vi "ROI Stand Alone Compatability check.vi"(8 "error in (no error)":errorcluster, 11 "Old ROI file path":path) -> (0 "error out":errorcluster, 1 "Proceed":bool, 3 "ROI file path (dup)":path, 5 "ROI fit info cluster":T1 {"ROI fit info"."Frame size"."Old" items=["100X100"=100, "128X128"=128, "200X200"=200, "256X256"=256, "512X512"=512, "1024x1024"=1024, "2048x2048"=2048]; "ROI fit info"."Frame size"."New" items=["100X100"=100, "128X128"=128, "200X200"=200, "256X256"=256, "512X512"=512, "1024x1024"=1024, "2048x2048"=2048]})   [LabVIEW 2017]
uses:
  Typedefs/ROI fitting info cluster.ctl
  Typedefs/Frame Size.ctl
  Typedefs/ROI ID Enum.ctl
  Typedefs/ROI management FG states.ctl
  <userlib>/My Palettes.lib/Files & paths/Spreadsheet/Read From Spreadsheet File (DBL)-Mod.vi
  Globals/gl_ROI Entry UI globals.vi
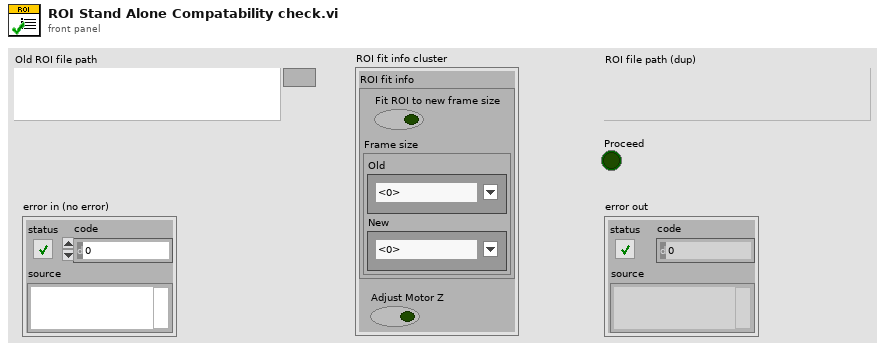
[diagram p1: front panel]
types:
  T1 = typedef "ROI fitting info cluster.ctl" = cluster{"ROI fit info":cluster{"Fit ROI to new frame size":bool, "Frame size":cluster{"Old":T2, "New":T2}}, "Adjust Motor Z":bool}
  T2 = typedef "Frame Size.ctl" = u16
  T3 = typedef "Fixed strings.ctl" = cluster{"ROI file name":string, "Normalised ROI file name":string, "Zplane Pockels values file name":string, "Functional data folder name":string, "Experiment Header file name":string, "Z-stack images folder name":string, "Groups setup rel. path":string, "Groups text file rel. path":string, "TDMS files folder name (F.img)":string, "TDMS files folder name (V.acq)":string, "TDMS files folder name (Pl.acq)":string, "Cycle rel times sequence file":string, "Dynamically called VIs folder name":string, "Time Series folder base name":string}
  T4 = typedef "ROI ID Enum.ctl" = enum16{"Point", "MiniScan", "Comp. MiniScan", "Rectangle", "Comp. volume", "Arb. plane point", "None"}
  T5 = typedef "ROI management FG states.ctl" = enum16{"Read", "Write", "Write-from dataset", "Clear Last", "Clear All", "Update ROIs time", "Reload last ROI set", "Offset all ROI", "Offset visible ROI"}
  T6 = enum8{"Enabled", "Disabled", "Disabled and Grayed Out"}
  T7 = typedef "ROI parameters data type.ctl" = cluster{"ROI index":dbl, "ROI ID":dbl, "ROI Time (ns)":dbl, "Pixels in ROI":dbl, "X start":dbl, "Y start":dbl, "Z start":dbl, "X stop":dbl, "Y stop":dbl, "Z stop":dbl, "Angle (deg)":dbl, "Composite ID":dbl, "Number of lines":dbl, "Frame Size":dbl, "Zoom":dbl, "Laser Power (%)":dbl, "ROI group ID":dbl, "Z Plane Idx":i32[], "Z Plane codes":i32[]}
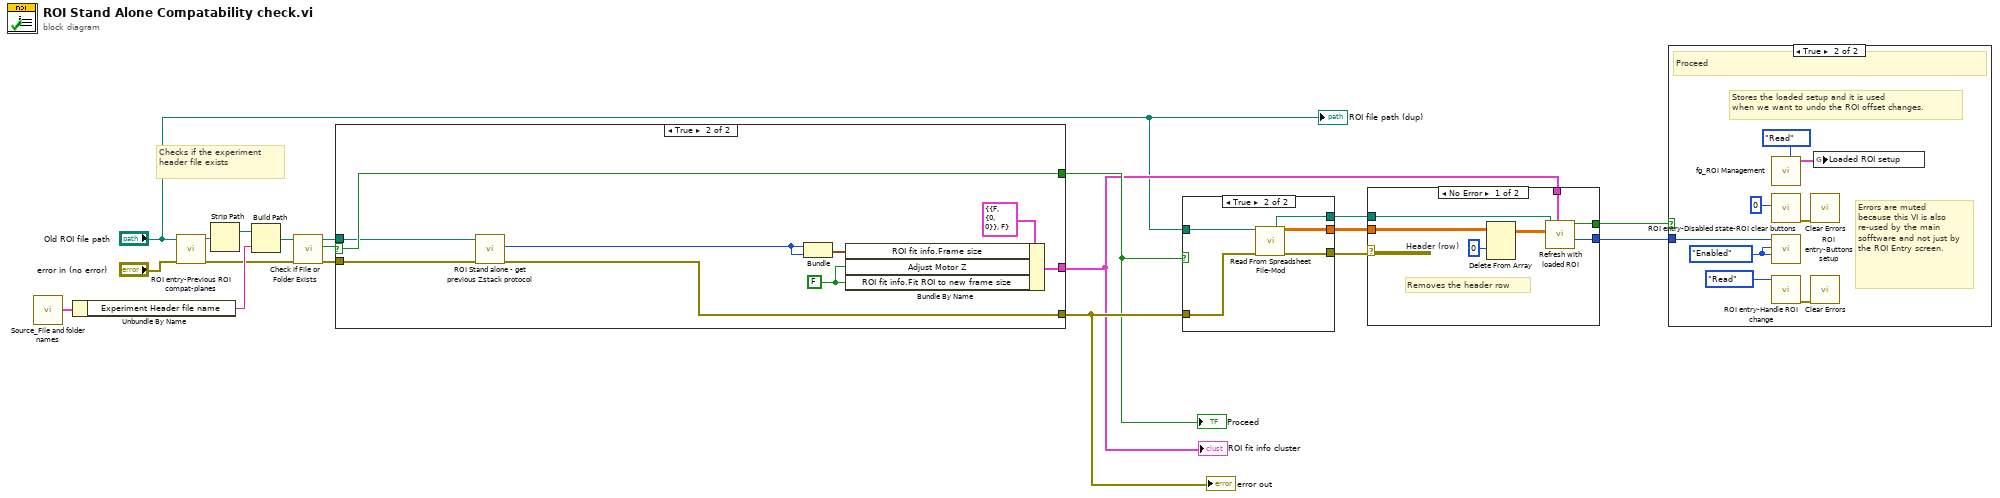
[diagram p0: block diagram]
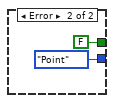
[diagram p3: hidden frame]
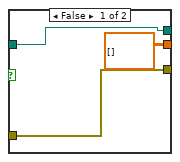
[diagram p4: hidden frame]
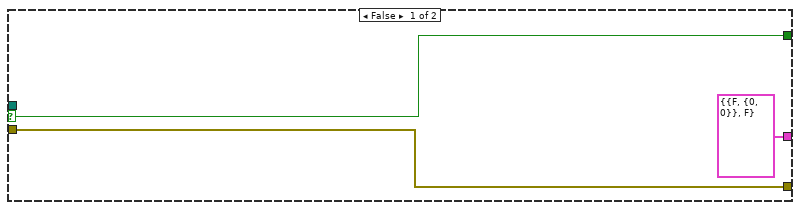
[diagram p5: hidden frame]
diagram:
  # "Checks if the experiment header file exists"
  n1 = call "Source_File and folder names.vi"() -> ("Fixed strings"=w17:T3)  [unwired: 1 in]
  n2 = Unbundle By Name(w17) -> ("Experiment Header file name"=w15:string)
  n3 = call "ROI entry-Previous ROI compat-planes.vi"("error in (no error)"="error in (no error)", "Old ROI file path"="Old ROI file path") -> ("error out"=w14:errorcluster, "Old ROI file path (dup)"=w13:path)  [unwired: 7 in, 1 out]
  n4 = Strip Path(path=w13) -> (stripped path=w16:path)  [unwired: 1 out]
  n5 = Build Path(base path=w16, name or relative path=w15) -> (appended path=w18:path)
  n6 = call <vilib>:"Check if File or Folder Exists.vi"("error in (no error)"=w14, "path"=w18) -> ("error out"=w11:errorcluster, "file or folder exists?"=w12:bool, "dup path"=w10:path)  [unwired: 7 in]
  n7 = case shown="True" w12 {
    selector: w12 -> [w22 w27]
    tunnel: w11 -> [w20 w26]
    tunnel: w10 -> [_ w25]
    tunnel: [T1 {"ROI fit info"={"Fit ROI to new frame size"=FALSE, "Frame size"={"Old"=0, "New"=0}}, "Adjust Motor Z"=FALSE} ("ROI fit info") w28] -> w4
    tunnel: [w22 w27] -> w8
    tunnel: [w20 w24] -> w9
    frame False {
    }
    frame True {
      w29 = FALSE ("Adjust Motor Z")
      n8 = call "ROI Stand alone - get previous Zstack protocol.vi"("error in (no error)"=w26, "path"=w25) -> ("error out"=w24:errorcluster, "Frame Size"=w23:T2)  [unwired: 5 in, 3 out]
      n9 = Bundle("Frame Size"=w23, "Frame Size"=w23) -> (w30:cluster{"Frame Size":T2, "Frame Size":T2})  [unwired: 1 in]
      n10 = Bundle By Name(cluster=T1 {"ROI fit info"={"Fit ROI to new frame size"=FALSE, "Frame size"={"Old"=0, "New"=0}}, "Adjust Motor Z"=FALSE} ("ROI fit info"), "ROI fit info.Frame size"=w30, "Adjust Motor Z"=w29, "ROI fit info.Fit ROI to new frame size"=w29) -> (w28:T1)
    }
  }
  "Proceed" <- w8
  "error out" <- w9
  "ROI fit info cluster" <- w4
  n11 = case shown="True" w8 {
    tunnel: w9 -> [w34 w39]
    tunnel: "Old ROI file path" -> [w32 w38]
    tunnel: [dbl[][] [] ("all rows") w37] -> w6
    tunnel: [w34 w36] -> w7
    tunnel: [w32 w35] -> w5
    frame False {
    }
    frame True {
      n12 = call-poly <userlib>:"Read From Spreadsheet File-Mod.vi"("file path (dialog if empty)"=w38, "error in"=w39) -> ("new file path (Not A Path if cancelled)"=w35:path, "all rows"=w37:dbl[][], "error out"=w36:errorcluster)  [unwired: 8 in, 3 out]
    }
  }
  n13 = case shown="No Error" w7 {
    tunnel: w6 -> [w45 _]
    tunnel: w5 -> [w44 _]
    tunnel: w4 -> [w43 _]
    tunnel: [w41 FALSE ("Proceed?")] -> w2
    tunnel: [w40 ROI_ID_Enum."Point" ("Last ROI Enum")] -> w3
    frame No Error {
      w46 = 0  # Header (row)
      # "Removes the header row"
      n14 = Delete From Array(array=w45, index (row)=w46) -> (array with subset deleted=w42:dbl[][])  [unwired: 2 in, 1 out]
      n15 = call "Refresh with loaded ROI.vi"("ROI fit info cluster"=w43, "Old ROI file's data"=w42, "Old ROI file path"=w44) -> ("Last ROI Enum"=w40:T4, "Proceed?"=w41:bool)  [unwired: 7 in]
    }
    frame Error {
    }
  }
  n16 = case shown="True" w2 {
    tunnel: w3 -> [_ w49]
    frame False {
      # "Do not proceed"
    }
    frame True {
      w50 = T6."Enabled" ("Done button disabled?")
      # "Stores the loaded setup and it is used\nwhen we want to undo the ROI offset changes."
      # "Errors are muted because this VI is also re-used by the main sofftware and not just by the ROI Entry screen."
      # "Proceed"
      n17 = call "fg_ROI Management.vi"("Function"=ROI_management_FG_states."Read") -> ("ROI Setup"=w51:T7[])  [unwired: 5 in, 5 out]
      n18 = call "ROI entry-Disabled state-ROI clear buttons.vi"("State"=0) -> ("error out"=w55:errorcluster)  [unwired: 10 in]
      n19 = call "ROI entry-Buttons setup.vi"("Acquisition button disabled?"=w50, "Done button disabled?"=w50, "ROI Enum"=w49) -> ()  [unwired: 9 in]
      n20 = call "ROI entry-Handle ROI change.vi"("ROI management"=ROI_management_FG_states."Read") -> ("error out"=w54:errorcluster)  [unwired: 8 in, 2 out]
      n21 = call <vilib>:"Clear Errors.vi"("error in (no error)"=w55) -> ()  [unwired: 5 in, 2 out]
      n22 = call <vilib>:"Clear Errors.vi"("error in (no error)"=w54) -> ()  [unwired: 5 in, 2 out]
      n23 = global write "gl_ROI Entry UI globals.vi" "Loaded ROI setup"(w51) -> ()
    }
  }
  "ROI file path (dup)" <- "Old ROI file path"
